vi "Watchdog Init.vi"(8 "error in (no error)":errorcluster, 11 "Number of Watchdogs":i32=1) -> (0 "error out":errorcluster)   [LabVIEW 2013, in "RT Watchdog.lvlib"]
uses:
  RT Watchdog.lvlib
  Watchdog actions.ctl
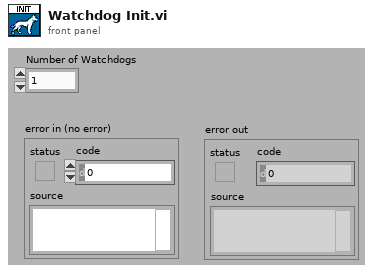
[diagram p1: front panel]
types:
  T1 = typedef "Watchdog actions.ctl" = enum16{"Init", "Enable", "Service", "Disable", "Check"}
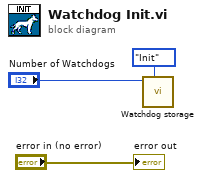
[diagram p0: block diagram]
diagram:
  n1 = call "Watchdog storage.vi"("Command"=Watchdog_actions."Init", "Number of Watchdogs"="Number of Watchdogs") -> ()  [unwired: 7 in, 3 out]
  "error out" <- "error in (no error)"
